vi "Untitled 1.vi"() -> ()   [LabVIEW 2013]
panel:
  out "floor(x/y)":u32
  out "x-y*floor(x/y)":u32
  in  "Puntos":u32
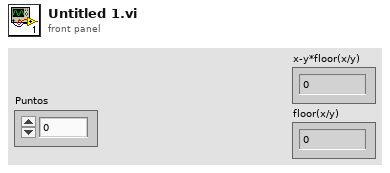
[diagram p1: front panel]
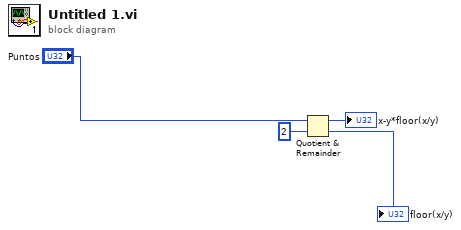
[diagram p0: block diagram]
diagram:
  n1 = Quotient & Remainder(x="Puntos", y=u32 2) -> (x-y*floor(x/y)=→"x-y*floor(x/y)":u32, floor(x/y)=→"floor(x/y)":u32)
